vi "Handling DO param.vi"(8 "error in (no error)":errorcluster, 9 "DO":bool[](array[boolean]), 10 "DOP":i32[][](array[numeric]), 11 "DO2D_def":bool[][](array[boolean])) -> (0 "error out":errorcluster, 3 "DO2D":bool[][](array[boolean]))   [LabVIEW 2019, in "Inputs.lvlib"]
uses:
  Inputs.lvlib
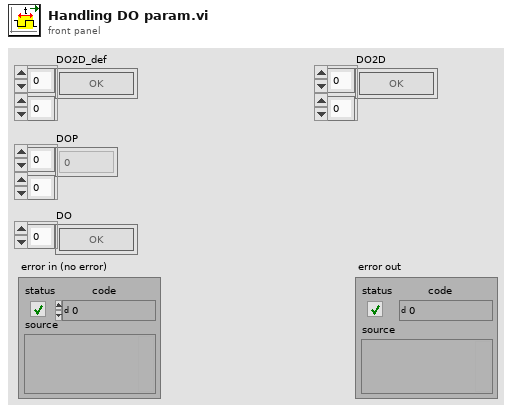
[diagram p1: front panel]
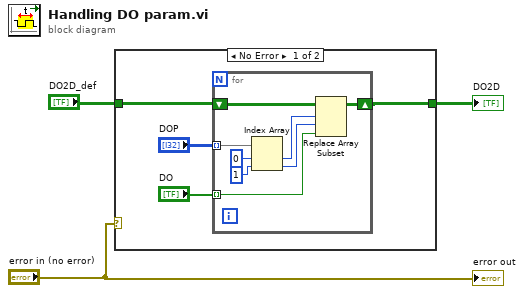
[diagram p0: block diagram]
diagram:
  n1 = case shown="No Error" "error in (no error)" {
    tunnel: [w6 w16] -> w1
    tunnel: "DO2D_def" -> [w7 w16]
    frame No Error {
      n2 = for {
        tunnel: "DOP" -> [w15] mode=indexing
        tunnel: "DO" -> [w11] mode=indexing
        shift-right: [w10] -> w6
        shift-left: w7 -> [w12]
        n3 = Index Array(array=w15, index #1=0 ("index (row)"), index #2=1 ("index (row)")) -> (element #1=w9:i32, element #2=w8:i32)
        n4 = Replace Array Subset(array=w12, new element=w11, index (row)=w9, index (col)=w8) -> (w10:bool[][])
      }
    }
    frame Error {
    }
  }
  "DO2D" <- w1
  "error out" <- "error in (no error)"
